vi "StationGlobals.vi"(8 "error in (no error)":errorcluster, 11 "Engine in":refnum<class "Engine.lvclass">) -> (0 "error out":errorcluster, 2 "StationGlobals":refnum<class "PropertyObject.lvclass">, 3 "Engine out":refnum<class "Engine.lvclass">)   [LabVIEW 2020, in "TSnax.lvlib" / "Engine.lvclass"]
uses:
  Engine.lvclass
  Engine.lvclass/Engine.ctl
  PropertyObject/PropertyObject.lvclass
  VariableContainer Type.ctl
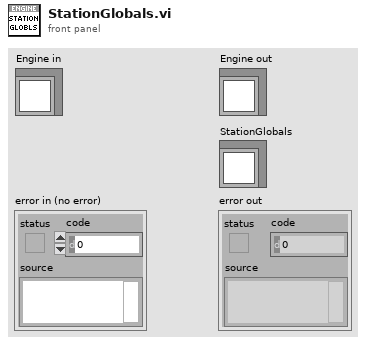
[diagram p1: front panel]
types:
  T1 = typedef "TSnax.lvlib/Engine.lvclass/Ref Data.ctl" = cluster{"Station Globals":refnum<class "PropertyObject.lvclass">, "Station Model":refnum<class "SequenceFile.lvclass">}
  T2 = typedef "TSnax.lvlib/Engine.lvclass/VariableContainer Type.ctl" = enum16{"StationGlobals", "TemporaryGlobals", "NewPropertyObject", "SubProperty"}
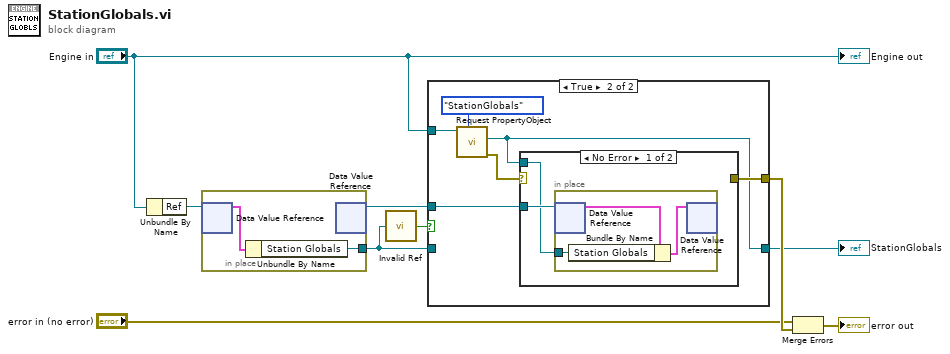
[diagram p0: block diagram]
diagram:
  n1 = Unbundle By Name("Engine in") -> ("Ref"=w7:refnum<data-value>)
  n2 = in-place {
    in-place-border: [w10] -> w4
    n3 = in-place-dvr #1(w7) -> (w11:T1)  [unwired: 1 out]
    n4 = Unbundle By Name(w11) -> ("Station Globals"=w10:refnum<class "PropertyObject.lvclass">)
    n5 = in-place-dvr #1() -> (w5:refnum<data-value>)  [unwired: 1 in, 1 out]
  }
  n6 = call "Invalid Ref.vi"("PropertyObject"=w4) -> ("Not a Valid Ref?"=w6:bool)
  n7 = case shown="True" w6 {
    tunnel: "Engine in" -> [_ w18]
    tunnel: w5 -> [_ w15]
    tunnel: w4 -> [w12 _]
    tunnel: [w12 w13] -> w2
    tunnel: [_ w14] -> w9
    frame False {
    }
    frame True {
      n8 = call "Request PropertyObject.vi"("Type"=VariableContainer_Type."StationGlobals", "Engine in"=w18) -> ("error out"=w16:errorcluster, "PropertyObject"=w13:refnum<class "PropertyObject.lvclass">)  [unwired: 8 in]
      n9 = case shown="No Error" w16 {
        selector: w16 -> [_ w24]
        tunnel: w13 -> [w19 _]
        tunnel: w15 -> [w20 _]
        tunnel: [_ w24] -> w14
        frame No Error {
          n10 = in-place {
            in-place-border: w19 -> [w21]
            n11 = in-place-dvr #2(w20) -> (w23:T1)  [unwired: 1 out]
            n12 = Bundle By Name(cluster=w23, "Station Globals"=w21) -> (w22:T1)
            n13 = in-place-dvr #2(w22) -> ()  [unwired: 2 out]
          }
        }
        frame Error {
        }
      }
    }
  }
  "StationGlobals" <- w2
  n14 = Merge Errors("error in (no error)", w9) -> (→"error out":errorcluster)
  "Engine out" <- "Engine in"
